vi "eec 10 final project.vi"() -> ()   [LabVIEW 2016]
uses:
  Program Files (x86)/National Instruments/LabVIEW 2016/examples/Instrument IO/Serial/support/Serial - Settings.ctl
  <vilib>/sound2/lvsound2.llb/Sound Data Format.ctl
  <vilib>/Instr/_visa.llb/VISA Configure Serial Port (Instr).vi
  <vilib>/sound2/lvsound2.llb/Sound File Write Open.vi
  <vilib>/sound2/lvsound2.llb/Sound File Write (DBL).vi
panel:
  out "Generated Sound File":path
  in  "Serial Settings":T1={"baud rate"=9600, "data bits"=8, "parity"=enum."None", "stop bits"=10, "flow control"=0} {"flow control" items=["None"=0, "XON/XOFF"=1, "RTS/CTS"=2, "DTR/DSR"=4]; "stop bits" items=["1.0"=10, "1.5"=15, "2.0"=20]; "data bits" min=5 max=8 step=1; "baud rate" items=["75"=75, "110"=110, "134"=134, "150"=150, "300"=300, "600"=600, "1200"=1200, "1800"=1800, "2400"=2400, "4800"=4800, "7200"=7200, "9600"=9600, "14400"=14400, "19200"=19200, "28800"=28800, "38400"=38400, "56000"=56000, "57600"=57600, "115200"=115200, "128000"=128000, "230400"=230400]}
  out "Elapsed Time (s)":dbl
  out "Index":i32
  out "Right Max":dbl
  out "Left Max":dbl
  out "Amplitude":dbl
  out "Angle":string
  in  "Time Delay (s)":dbl
  out "Combined":dynamicdata(graph) caption="Total Signal"
  out "Combined - Filtered":dynamicdata(graph) caption="Filtered Total Signal"
  in  "Stop":bool
  in  "Record":bool
  in  "Volume":dbl(slide)=0.125 scale=0.0..1.0
  in  "Bass":dbl(slide)=0.4693877551020408 scale=0.0..1.0
  in  "Midtone":dbl(slide)=0.4081632653061224 scale=0.0..1.0
  in  "Treble":dbl(slide)=0.4081632653061224 scale=0.0..1.0
  out "Right Plot":dynamicdata(graph)
  out "Left Plot":dynamicdata(graph)
  in  "VISA resource name":refnum<visa-resource-name>="COM1"
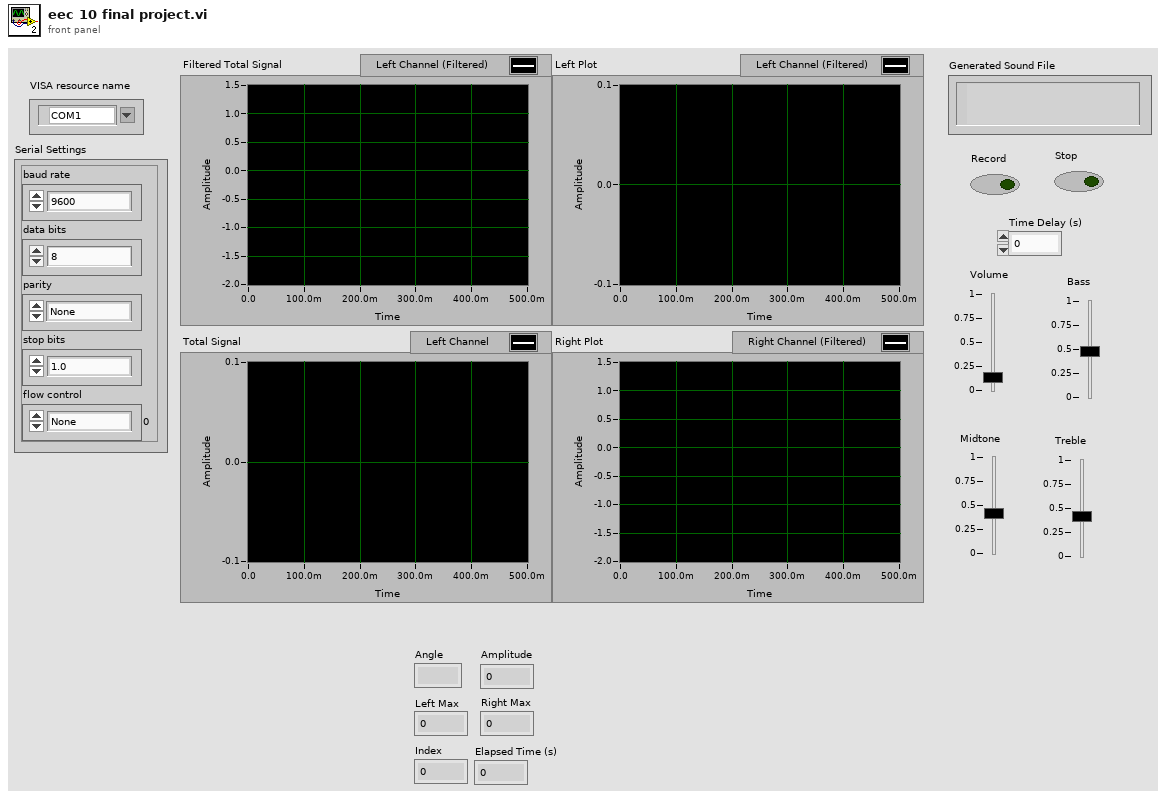
[diagram p1: front panel]
types:
  T1 = typedef "Serial - Settings.ctl" = cluster{"baud rate":u32, "data bits":u16, "parity":enum16{"None", "Odd", "Even", "Mark", "Space"}, "stop bits":u16, "flow control":u16}
  T2 = typedef "Sound Data Format.ctl" = cluster{"sample rate (S/s)":dbl, "number of channels":i32, "bits per sample":i32}
  T3 = typedef "Sound File Refnum.ctl" = refnum<file>
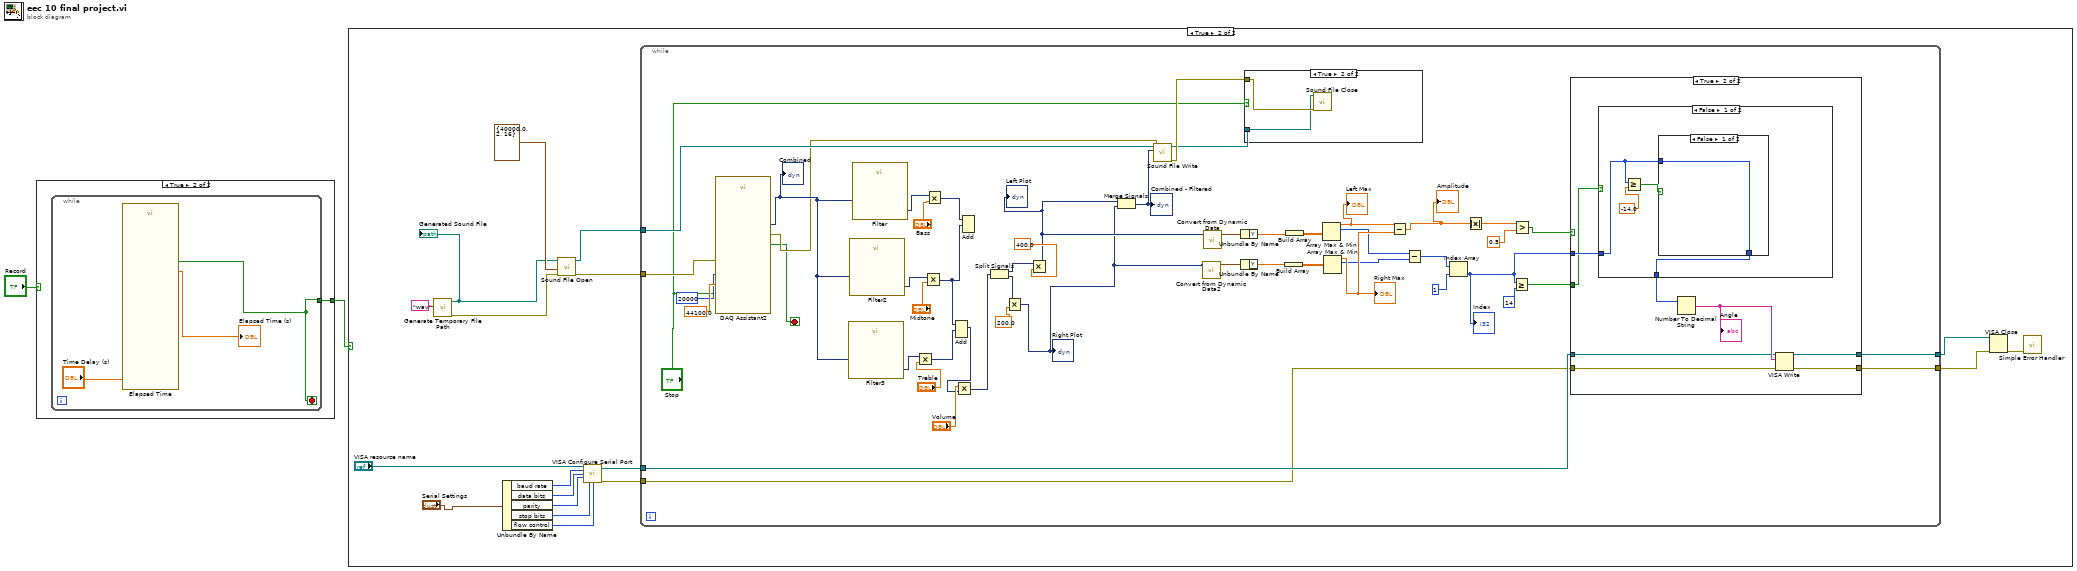
[diagram p0: block diagram]
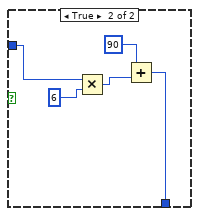
[diagram p5: hidden frame]
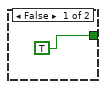
[diagram p7: hidden frame]
diagram:
  n1 = case shown="True" "Record" {
    tunnel: [TRUE w4] -> w1
    frame False {
    }
    frame True {
      n2 = while {
        tunnel: [w5] -> w4
        stop <- w5 stop-if-true
        n3 = call "Elapsed Time"("Time Target (s)"="Time Delay (s)") -> ("Elapsed Time (s)"=→"Elapsed Time (s)":dbl, "Time has Elapsed"=w5:bool)  [unwired: 11 in, 6 out]
      }
    }
  }
  n4 = case shown="True" w1 {
    frame False {
    }
    frame True {
      n5 = call <vilib>:"Generate Temporary File Path.vi"("Temporary File Extension (tmp)"="wav") -> ("error out"=w8:errorcluster, "Unique Temporary File Path"=w9:path)  [unwired: 9 in]
      "Generated Sound File" <- w9
      n6 = Unbundle By Name("Serial Settings") -> ("baud rate"=w24:u32, "data bits"=w23:u16, "parity"=w22:enum16{"None", "Odd", "Even", "Mark", "Space"}, "stop bits"=w21:u16, "flow control"=w20:u16)
      n7 = call-poly <vilib>:"Sound File Open.vi"("error in (no error)"=w8, "sound format"=T2 {"sample rate (S/s)"=40000.0, "number of channels"=2, "bits per sample"=16} ("Sound Format"), "path"=w9) -> ("error out"=w19:errorcluster, "sound file refnum"=w18:T3)  [unwired: 7 in]
      n8 = call-poly "VISA Configure Serial Port"("VISA resource name"="VISA resource name", "baud rate (9600)"=w24, "data bits (8)"=w23, "parity (0:none)"=w22, "stop bits (10: 1 bit)"=w21, "flow control (0:none)"=w20) -> ("VISA resource name out"=w17:refnum<visa-resource-name>, "error out"=w16:errorcluster)  [unwired: 3 in, 5 out]
      n9 = while {
        tunnel: w19 -> [w32]
        tunnel: w18 -> [w33]
        tunnel: w17 -> [w37]
        tunnel: w16 -> [w36]
        tunnel: [w35] -> w15
        tunnel: [w34] -> w14
        stop <- w29 stop-if-true
        n10 = call "DAQ Assistant2"("rate"=44100.0, "number of samples"=20000, "error in"=w32, "stop (F)"="Stop") -> ("data"=w31:dynamicdata, "stopped"=w29:bool, "error out"=w30:errorcluster)  [unwired: 12 in, 1 out]
        "Combined" <- w31
        n11 = call "Filter3"("Signal"=w31) -> ("Filtered Signal"=w75:dynamicdata)  [unwired: 9 in, 1 out]
        n12 = call "Filter2"("Signal"=w31) -> ("Filtered Signal"=w76:dynamicdata)  [unwired: 9 in, 1 out]
        n13 = call "Filter"("Signal"=w31) -> ("Filtered Signal"=w77:dynamicdata)  [unwired: 9 in, 1 out]
        n14 = Multiply(x=w75, y="Treble") -> (x*y=w69:dynamicdata)
        n15 = Multiply(x=w76, y="Midtone") -> (x*y=w70:dynamicdata)
        n16 = Multiply(x=w77, y="Bass") -> (x*y=w71:dynamicdata)
        n17 = Add(1:w69, 2:w70) -> (0:w66:dynamicdata)  [unwired: 1 in, 1 out]
        n18 = Multiply(x="Volume", y=w66) -> (x*y=w67:dynamicdata)
        n19 = Add(1:w70, 2:w71) -> ()  [unwired: 1 in, 2 out]
        n20 = Split Signals(w67) -> (w63:dynamicdata, w65:dynamicdata)  [unwired: 2 in]
        n21 = Multiply(x=w65, y=200.0) -> (x*y=w59:dynamicdata)
        "Right Plot" <- w59
        n22 = Multiply(x=w63, y=400.0) -> (x*y=w60:dynamicdata)
        "Left Plot" <- w60
        n23 = Merge Signals(w60, w59) -> (w61:dynamicdata)
        "Combined - Filtered" <- w61
        n24 = call-poly <vilib>:"Sound File Write.vi"("error in (no error)"=w30, "data"=w61, "sound file refnum"=w33) -> ("error out"=w39:errorcluster, "sound file refnum out"=w38:T3)  [unwired: 7 in]
        n25 = call "Convert from Dynamic Data2"("Dynamic Data Type"=w59) -> ("Waveform"=w58:waveform(dbl))  [unwired: 3 in]
        n26 = call "Convert from Dynamic Data"("Dynamic Data Type"=w60) -> ("Waveform"=w57:waveform(dbl))  [unwired: 3 in]
        n27 = Unbundle By Name(w57) -> ("Y"=w55:dbl[])
        n28 = Unbundle By Name(w58) -> ("Y"=w56:dbl[])
        n29 = case shown="True" "Stop" {
          tunnel: w39 -> [_ w79]
          tunnel: w38 -> [_ w78]
          frame False {
          }
          frame True {
            n30 = call <vilib>:"Sound File Close.vi"("error in (no error)"=w79, "sound file refnum"=w78) -> ()  [unwired: 9 in, 1 out]
          }
        }
        n31 = Build Array(w56) -> (w53:dbl[][])
        n32 = Build Array(w55) -> (w54:dbl[][])
        n33 = Array Max & Min(array=w54) -> (max value=w52:dbl, max index (indices)=w49:i32[])  [unwired: 2 out]
        "Left Max" <- w52
        n34 = Array Max & Min(array=w53) -> (max value=w51:dbl, max index (indices)=w50:i32[])  [unwired: 2 out]
        "Right Max" <- w51
        n35 = Subtract(x=w52, y=w51) -> (x-y=w48:dbl)
        "Amplitude" <- w48
        n36 = Subtract(x=w49, y=w50) -> (x-y=w47:i32[])
        n37 = Index Array(array=w47, index=1) -> (element=w40:i32)
        "Index" <- w40
        n38 = Absolute Value(x=w48) -> (abs(x)=w44:dbl)
        n39 = Greater Or Equal?(x=w40, y=14) -> (x >= y?=w41:bool)
        n40 = Greater?(x=w44, y=0.5) -> (0:w42:bool)
        n41 = case shown="True" w42 {
          tunnel: w41 -> [_ w88]
          tunnel: w40 -> [_ w89]
          tunnel: w37 -> [w81 w85]
          tunnel: w36 -> [w80 w84]
          tunnel: [w81 w83] -> w35
          tunnel: [w80 w82] -> w34
          frame False {
          }
          frame True {
            n42 = case shown="False" w88 {
              tunnel: w89 -> [w92 w100]
              tunnel: [w90 w100] -> w87
              frame False {
                n43 = Greater Or Equal?(x=w92, y=-14.0) -> (x >= y?=w91:bool)
                n44 = case shown="False" w91 {
                  tunnel: w92 -> [w94 w97]
                  tunnel: [w94 w99] -> w90
                  frame False {
                  }
                  frame True {
                    n45 = Multiply(x=w97, y=6) -> (x*y=w95:i32)
                    n46 = Add(x=90, y=w95) -> (x+y=w99:i32)
                  }
                }
              }
              frame True {
              }
            }
            n47 = Number To Decimal String(number=w87) -> (decimal integer string=w86:string)  [unwired: 1 in]
            "Angle" <- w86
            n48 = VISA Write(VISA resource name=w85, write buffer=w86, error in (no error)=w84) -> (VISA resource name out=w83:refnum<visa-resource-name>, error out=w82:errorcluster)  [unwired: 1 out]
          }
        }
      }
      n49 = VISA Close(VISA resource name=w15, error in (no error)=w14) -> (error out=w13:errorcluster)
      n50 = call <vilib>:"Simple Error Handler.vi"("error in (no error)"=w13) -> ()  [unwired: 4 in, 5 out]
    }
  }
